vi "Set Ctl Picture.vi"() -> ()   [LabVIEW 2020, in "VolatusGUIElements.lvlib" / "2WayValveH.lvclass"]
uses:
  2WayValveH.lvclass
  Values.ctl
  Channel State.ctl
  Unused Element.ctl
  Command Picture.vi
  Feedback Picture.vi
  Energized Picture.vi
  2WayValveH.lvclass/2WayValveH.ctl
panel:
  out "error out":errorcluster
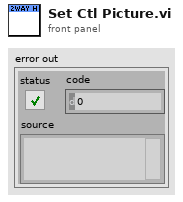
[diagram p1: front panel]
types:
  T1 = typedef "VolatusGUIElements.lvlib/2WayValveH.lvclass/Values.ctl" = cluster{"Command":T2, "CmdFB":T2, "Closed":T2, "Open":T2, "Energized":T2}
  T2 = typedef "VolatusGUIElements.lvlib/2WayValveH.lvclass/Channel State.ctl" = cluster{"Value":bool, "Stale":bool, "Config":bool, "Error":bool, "Prev":bool}
  T3 = typedef "VolatusGUIElements.lvlib/2WayValveH.lvclass/Unused Element.ctl" = cluster{"Command":bool, "Feedback":bool, "Energized":bool}
  T4 = typedef "VolatusGUIElements.lvlib/2WayValveH.lvclass/Valve Pictures.ctl" = cluster{"Command":T5, "Feedback":T7, "Energized":T8}
  T5 = typedef "VolatusGUIElements.lvlib/2WayValveH.lvclass/Command Pictures.ctl" = cluster{"Error":T6, "Config":T6, "Stale":T6, "Close":T6, "Open":T6, "TranClose":T6, "TranOpen":T6}
  T6 = typedef "VolatusGUIElements.lvlib/2WayValveH.lvclass/Picture.ctl" = enum16{"Blank", "OutClose", "OutOpen", "OutTranClose", "OutTranOpen", "OutConfig", "OutStale", "OutError", "InClose", "InOpen", "InTranClose", "InTranOpen", "InConfig", "InStale", "InError", "EnOff", "EnOn", "EnConfig", "EnStale", "EnError"}
  T7 = typedef "VolatusGUIElements.lvlib/2WayValveH.lvclass/Feedback Pictures.ctl" = cluster{"Error":T6, "Config":T6, "Stale":T6, "Closed":T6, "Open":T6, "TranClose":T6, "TranOpen":T6}
  T8 = typedef "VolatusGUIElements.lvlib/2WayValveH.lvclass/Energized Pictures.ctl" = cluster{"Error":T6, "Config":T6, "Stale":T6, "False":T6, "True":T6}
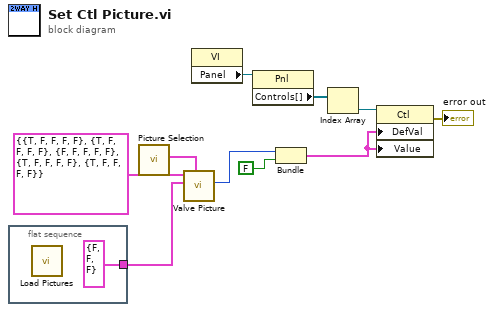
[diagram p0: block diagram]
diagram:
  n1 = flat-sequence {
    tunnel: [T3 {"Command"=FALSE, "Feedback"=FALSE, "Energized"=FALSE} ("Unused Element")] -> w5
    frame #0 {
      n2 = call "Load Pictures.vi"() -> ()  [unwired: 11 in, 1 out]
    }
  }
  n3 = call "Picture Selection.vi"() -> ("Valve Pictures"=w7:T4)  [unwired: 11 in]
  n4 = call "Valve Picture.vi"("Valve Pictures"=w7, "Unused Element"=w5, "Values"=T1 {"Command"={"Value"=TRUE, "Stale"=FALSE, "Config"=FALSE, "Error"=FALSE, "Prev"=FALSE}, "CmdFB"={"Value"=TRUE, "Stale"=FALSE, "Config"=FALSE, "Error"=FALSE, "Prev"=FALSE}, "Closed"={"Value"=FALSE, "Stale"=FALSE, "Config"=FALSE, "Error"=FALSE, "Prev"=FALSE}, "Open"={"Value"=TRUE, "Stale"=FALSE, "Config"=FALSE, "Error"=FALSE, "Prev"=FALSE}, "Energized"={"Value"=TRUE, "Stale"=FALSE, "Config"=FALSE, "Error"=FALSE, "Prev"=FALSE}}) -> ("Feedback Picture"=w4:T6)  [unwired: 6 in, 2 out]
  n5 = property class="VI"() -> ("Panel"=w10:refnum<vi>)  [unwired: 2 in, 2 out]
  n6 = property class="Pnl"(reference=w10) -> ("Controls[]"=w9:refnum<vi>[])  [unwired: 1 in, 2 out]
  n7 = Bundle("Feedback Picture"=w4, FALSE) -> (w1:cluster{"Feedback Picture":T6, bool})  [unwired: 1 in]
  n8 = Index Array(array=w9) -> (element=w8:refnum<vi>)  [unwired: 1 in]
  n9 = property class="Ctl"(reference=w8, "DefVal"=w1, "Value"=w1) -> (error out=→"error out":errorcluster)  [unwired: 1 in, 1 out]
